vi "LED_Set.vi"(8 "error in (no error)":errorcluster caption="错误输入（无错误）", 9 "board PF R":bool[](array[boolean]), 10 "board PF L":bool[](array[boolean]), 11 "组合框":string(combo)) -> (0 "error out":errorcluster caption="错误输出", 3 "连接的字符串":string)   [LabVIEW 2018]
uses:
  Subvi/Global.vi
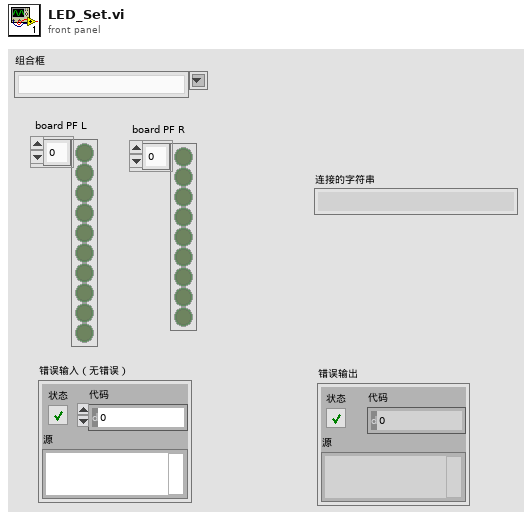
[diagram p1: front panel]
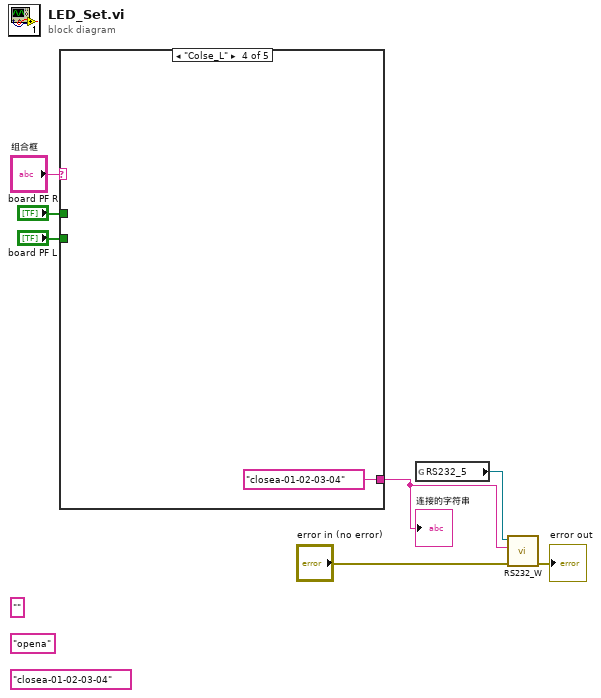
[diagram p0: block diagram]
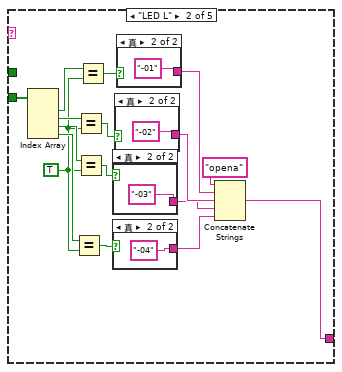
[diagram p3: hidden frame]
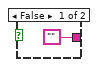
[diagram p4: hidden frame]
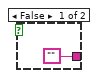
[diagram p5: hidden frame]
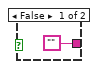
[diagram p6: hidden frame]
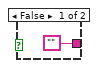
[diagram p7: hidden frame]
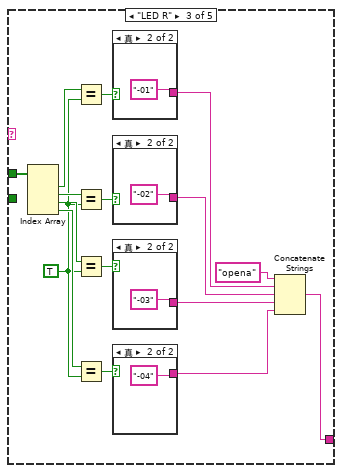
[diagram p8: hidden frame]
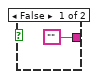
[diagram p9: hidden frame]
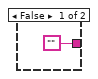
[diagram p10: hidden frame]
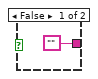
[diagram p11: hidden frame]
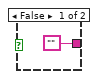
[diagram p12: hidden frame]
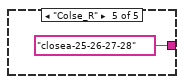
[diagram p13: hidden frame]
diagram:
  (unwired) "opena" ("字符串")
  (unwired) "closea-01-02-03-04"
  (unwired) ""
  n1 = case shown="\"Colse_L\"" "组合框" {
    tunnel: "board PF L" -> [_ w23 _ _ _]
    tunnel: [_ w9 w34 "closea-01-02-03-04" "closea-25-26-27-28"] -> w3
    tunnel: "board PF R" -> [_ _ w32 _ _]
    frame "假", Default {
    }
    frame "LED L" {
      w14 = TRUE
      n2 = Index Array(array=w23) -> (element #1=w22:bool, element #2=w21:bool, element #3=w20:bool, element #4=w19:bool)  [unwired: 4 in]
      n3 = Equal?(x=w19, y=w14) -> (x = y?=w15:bool)
      n4 = Equal?(x=w21, y=w14) -> (x = y?=w17:bool)
      n5 = Equal?(x=w20, y=w14) -> (x = y?=w16:bool)
      n6 = Equal?(x=w22, y=w14) -> (x = y?=w18:bool)
      n7 = case shown="真" w16 {
        tunnel: ["" "-03"] -> w11
        frame False {
        }
        frame True {
        }
      }
      n8 = case shown="真" w15 {
        tunnel: ["" "-04"] -> w10
        frame False {
        }
        frame True {
        }
      }
      n9 = case shown="真" w17 {
        tunnel: ["" "-02"] -> w12
        frame False {
        }
        frame True {
        }
      }
      n10 = case shown="真" w18 {
        tunnel: ["" "-01"] -> w13
        frame False {
        }
        frame True {
        }
      }
      n11 = Concatenate Strings("opena" ("字符串"), w13, w12, w11, w10) -> (w9:string)
    }
    frame "LED R" {
      w39 = TRUE
      n12 = Index Array(array=w32) -> (element #1=w47:bool, element #2=w46:bool, element #3=w45:bool, element #4=w44:bool)  [unwired: 4 in]
      n13 = Equal?(x=w47, y=w39) -> (x = y?=w43:bool)
      n14 = Equal?(x=w46, y=w39) -> (x = y?=w42:bool)
      n15 = Equal?(x=w45, y=w39) -> (x = y?=w41:bool)
      n16 = Equal?(x=w44, y=w39) -> (x = y?=w40:bool)
      n17 = case shown="真" w43 {
        tunnel: ["" "-01"] -> w38
        frame False {
        }
        frame True {
        }
      }
      n18 = case shown="真" w42 {
        tunnel: ["" "-02"] -> w37
        frame False {
        }
        frame True {
        }
      }
      n19 = case shown="真" w41 {
        tunnel: ["" "-03"] -> w36
        frame False {
        }
        frame True {
        }
      }
      n20 = case shown="真" w40 {
        tunnel: ["" "-04"] -> w35
        frame False {
        }
        frame True {
        }
      }
      n21 = Concatenate Strings("opena" ("字符串"), w38, w37, w36, w35) -> (w34:string)
    }
    frame "Colse_L" {
    }
    frame "Colse_R" {
    }
  }
  "连接的字符串" <- w3
  n22 = global read "Global.vi" "RS232_5"() -> (w4:refnum<visa-resource-name>)
  n23 = call "RS232_W.vi"("error in (no error)"="error in (no error)", "CMD"=w3, "VISA资源名称"=w4) -> ("error out"=→"error out":errorcluster)  [unwired: 6 in, 2 out]
